vi "Generate output.vi"(8 "error in (no error)":errorcluster, 10 "First call":bool, 11 "Software Lock-in in":refnum<class "Software Lock-in.lvclass">) -> (0 "error out":errorcluster, 2 "Sine wave":dbl[](array[numeric]), 3 "Software Lock-in out":refnum<class "Software Lock-in.lvclass">)   [LabVIEW 2015, in "Software Lock-in.lvclass"]
uses:
  Software Lock-in.lvclass
  Software Lock-in.lvclass/Software Lock-in.ctl
  <vilib>/Analysis/NI_AALBase.lvlib
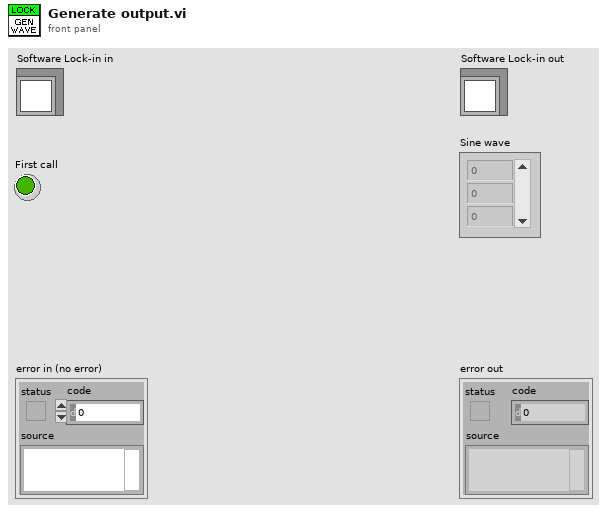
[diagram p1: front panel]
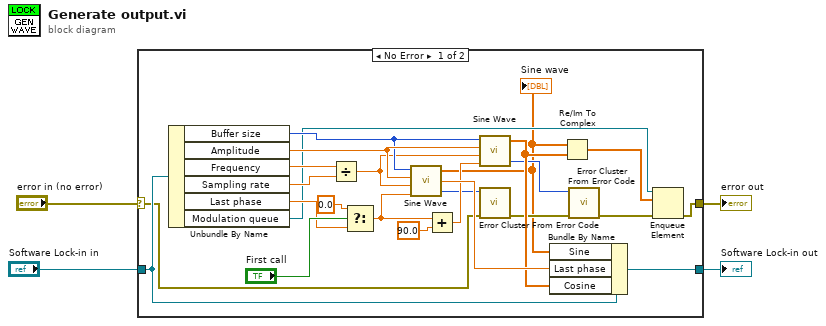
[diagram p0: block diagram]
diagram:
  n1 = case shown="No Error" "error in (no error)" {
    selector: "error in (no error)" -> [w7 w30]
    tunnel: [w6 w30] -> w3
    tunnel: [w28 w29] -> w1
    tunnel: "Software Lock-in in" -> [w26 w29]
    frame No Error {
      n2 = Unbundle By Name(w26) -> ("Buffer size"=w19:i32, "Amplitude"=w25:dbl, "Frequency"=w23:dbl, "Sampling rate"=w15:dbl, "Last phase"=w17:dbl, "Modulation queue"=w13:refnum<queue>)
      n3 = Divide(x=w23, y=w15) -> (x/y=w16:dbl)
      n4 = Select(t=0.0, s="First call", f=w17) -> (s? t:f=w22:dbl)
      n5 = call <vilib>:"Sine Wave.vi"("samples"=w19, "amplitude"=w25, "frequency"=w16, "phase in"=w22) -> ("sine wave"=w5:dbl[], "phase out"=w27:dbl, "error"=w11:i32)  [unwired: 1 in]
      "Sine wave" <- w5
      n6 = Add(x=w22, y=90.0) -> (x+y=w20:dbl)
      n7 = call <vilib>:"Sine Wave.vi"("samples"=w19, "amplitude"=w25, "frequency"=w16, "phase in"=w20) -> ("sine wave"=w14:dbl[], "error"=w9:i32)  [unwired: 1 in, 1 out]
      n8 = call <vilib>:"Error Cluster From Error Code.vi"("error in (no error)"=w7, "error code (0)"=w11) -> ("error out"=w10:errorcluster)  [unwired: 7 in]
      n9 = Bundle By Name(cluster=w26, "Sine"=w5, "Last phase"=w27, "Cosine"=w14) -> (w28:refnum<class "Software Lock-in.lvclass">)
      n10 = Re/Im To Complex(1:w14, 2:w5) -> (0:w12:cdb[])
      n11 = call <vilib>:"Error Cluster From Error Code.vi"("error in (no error)"=w10, "error code (0)"=w9) -> ("error out"=w8:errorcluster)  [unwired: 7 in]
      n12 = Enqueue Element(queue=w13, element=w12, error in (no error)=w8) -> (error out=w6:errorcluster)  [unwired: 1 in, 2 out]
    }
    frame Error {
    }
  }
  "error out" <- w3
  "Software Lock-in out" <- w1
